vi "TL4000 Set Temperature Setpoint Limits.vi"(8 "error in (no error)":errorcluster {"code" format="%.0x"}, 9 "Setpoint High Limit (50.0)":dbl=50.0, 10 "Setpoint Low Limit (0.0)":dbl, 11 "instrument handle":refnum<visa-resource-name>) -> (0 "error out":errorcluster {"code" format="%.0x"}, 3 "instrument handle out":refnum<visa-resource-name>)   [LabVIEW 2019]
doc: "This VI sets the user defined temperature setpoint limits.\n\nNote: \nThis VI is valid for: TED4000, ITC4000, CLD1000"
uses:
  TL4000_32.dll
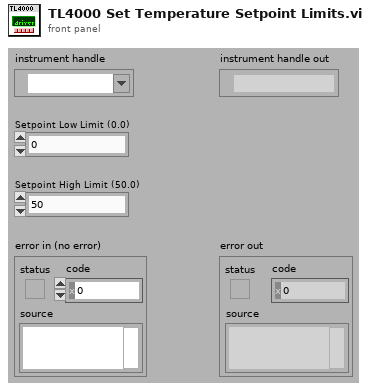
[diagram p1: front panel]
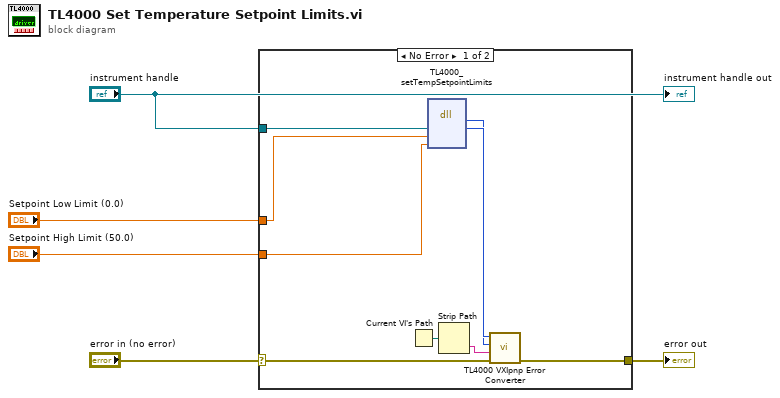
[diagram p0: block diagram]
diagram:
  n1 = case shown="No Error" "error in (no error)" {
    selector: "error in (no error)" -> [w9 w15]
    tunnel: [w8 w15] -> w5
    tunnel: "instrument handle" -> [w13 _]
    tunnel: "Setpoint Low Limit (0.0)" -> [w7 _]
    tunnel: "Setpoint High Limit (50.0)" -> [w6 _]
    frame No Error {
      n2 = Current VI's Path() -> (path=w14:path)
      n3 = dll-call lib="TL4000_32.*" fn="TL4000_setTempSetpointLimits"("Instrument Handle"=w13, "Setpoint Low Limit"=w7, "Setpoint High Limit"=w6) -> (w11:i32, "Instrument Handle"=w12:u32)  [unwired: 5 in, 2 out]
      n4 = Strip Path(path=w14) -> (name=w10:string)  [unwired: 1 out]
      n5 = call "TL4000 VXIpnp Error Converter.vi"("error in (no error)"=w9, "Name Of VI (\"\")"=w10, "CVI Error Code (0)"=w11, "instrument handle"=w12) -> ("error out"=w8:errorcluster)  [unwired: 6 in, 1 out]
    }
    frame Error {
    }
  }
  "error out" <- w5
  "instrument handle out" <- "instrument handle"
